vi "Test.vi"() -> ()   [LabVIEW 2019, in "Test.lvlib"]
doc: "This template is for the Queued Message Handler design pattern.\n\nThe Event Handling Loop generates messages based on user interface actions.\n\nThe Message Handling Loop processes messages generated by the Event Handling Loop, or by other messages. The messages are string values, so new messages can be added easily to the Message Cases case structure in the Message Handling Loop. Each message cluster can also provide an optional value for Message Data, which is a variant that can be converted to whatever message-specific data is required.a"
uses:
  Test.lvlib
  Data.ctl
  Message Queue/State Name.ctl
  Support/Message Queue/State Name.ctl
  <vilib>/event_ctls.llb/usereventprio.ctl
  0c61461a-fa07-4497-8c8c-8d3ef654e9c8.vi
  bad579f2-958a-4e04-a1a5-1778729f7708.vi
  681f6a39-68c9-4eb8-ab39-fd2fc03f9966.vi
  <vilib>/Utility/error.llb/Clear Errors.vi
  Message Queue/Enqueue (Single).vi
  <vilib>/Utility/error.llb/Error Cluster From Error Code.vi
  Message Queue/Enqueue (Array).vi
  Support/Message Queue/Reference Queue.vi
  <vilib>/ErrorRing/Error Ring.xnode
  Support/Message Queue/Message Queue.lvlib
panel:
  out "Headline":string
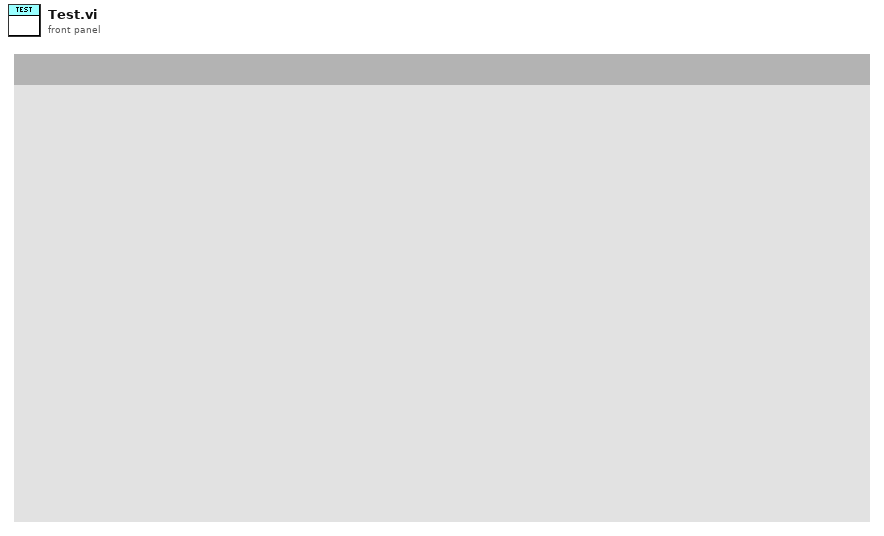
[diagram p1: front panel]
types:
  T1 = typedef "Test.lvlib/State Name.ctl" = enum16{"Default", "Initialize", "Re-Initialize", "Initialize Data", "Initialize Panel", "[Event Structure] Update Data", "Error", "Exit"}
  T2 = typedef "Test.lvlib/Data.ctl" = cluster{"Exit":bool, "States":T1}
  T3 = typedef "Message Queue Ref.ctl" = refnum<queue>
  T4 = typedef "Message Queue.lvlib/State Name.ctl" = enum16{"Default", "Initialize", "Initialize Data", "Initialize Modules", "Initialize Panel", "Close FP", "Open FP", "Initialize Menu", "Mode", "Update Subpanel", "Error", "Open Help", "About", "Open WebResources", "Exit"}
  T5 = typedef "usereventprio.ctl" = enum32{"high priority", "normal priority"}
  T6 = cluster{"Call Chain":string[], "Custom State Name":string, "timed out?":bool}
  T7 = enum16{"Left Button", "Center Button", "Right Button", "Window Close"}
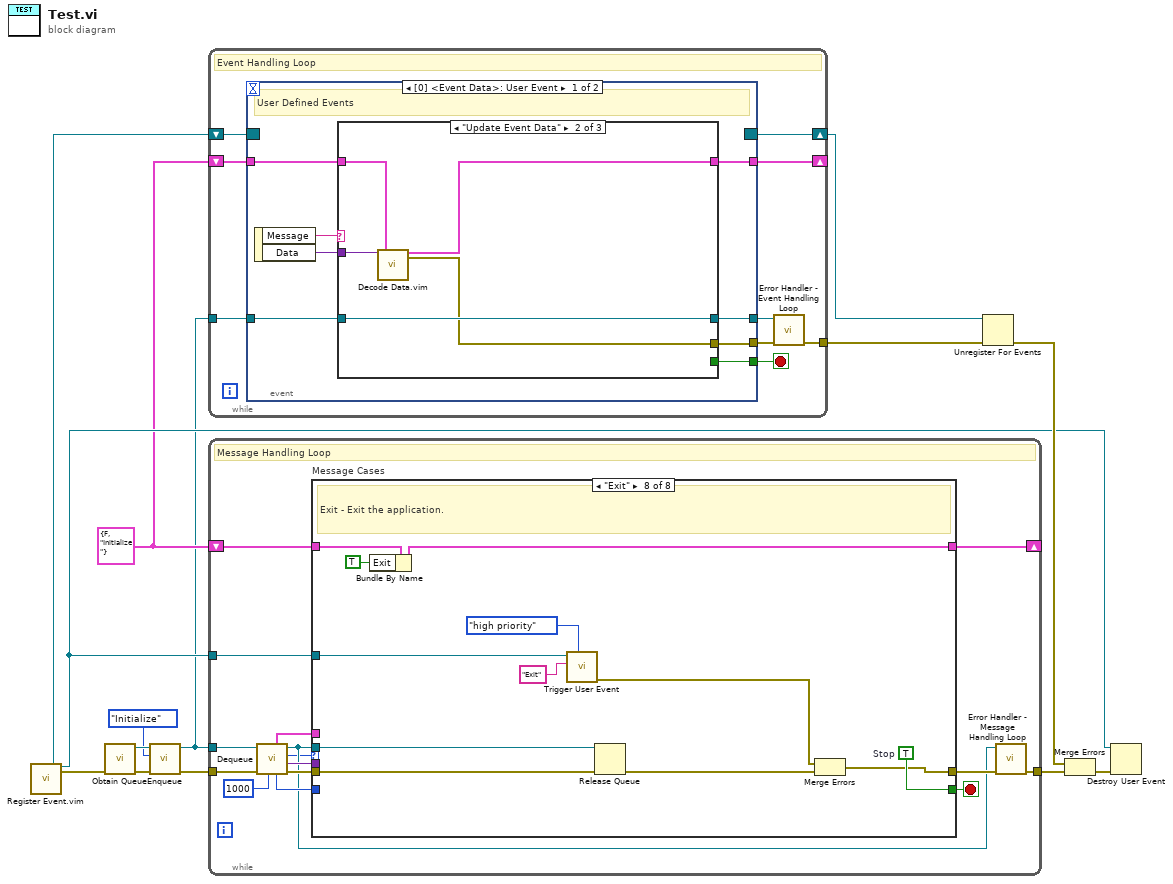
[diagram p0: block diagram]
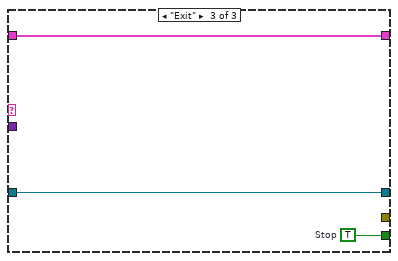
[diagram p3: hidden frame]
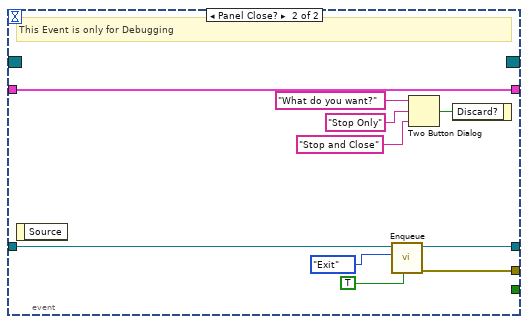
[diagram p4: hidden frame]
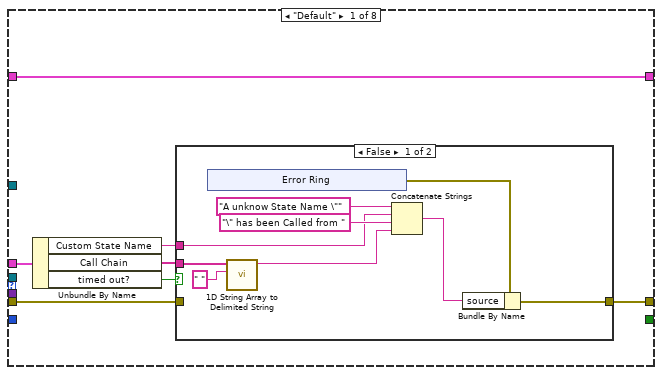
[diagram p5: hidden frame]
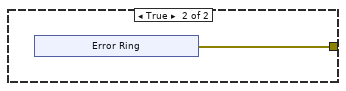
[diagram p6: hidden frame]
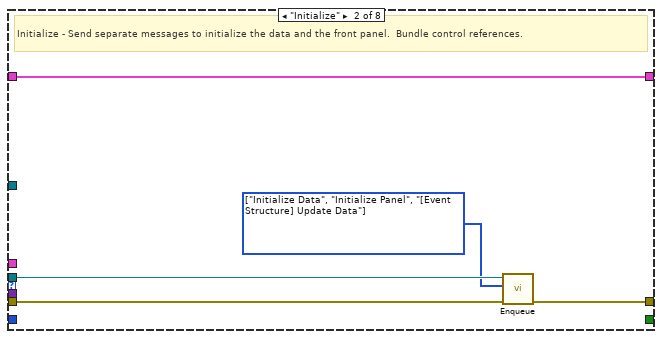
[diagram p7: hidden frame]
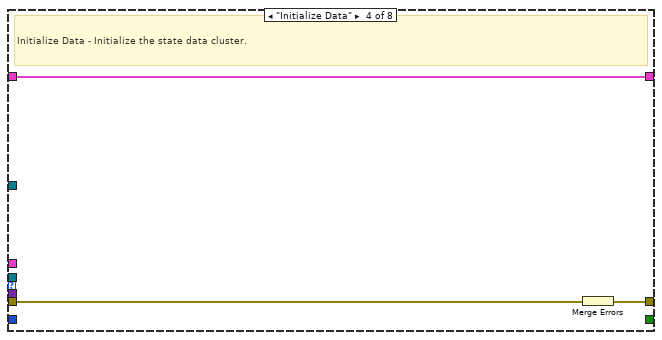
[diagram p9: hidden frame]
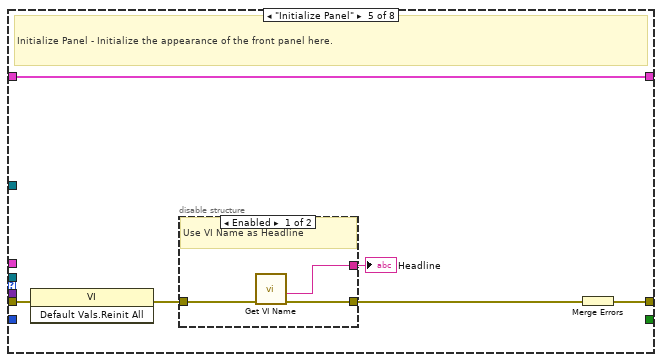
[diagram p10: hidden frame]
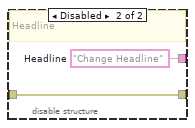
[diagram p11: hidden frame]
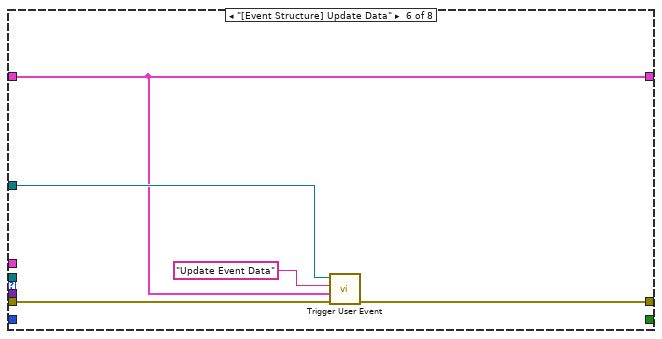
[diagram p12: hidden frame]
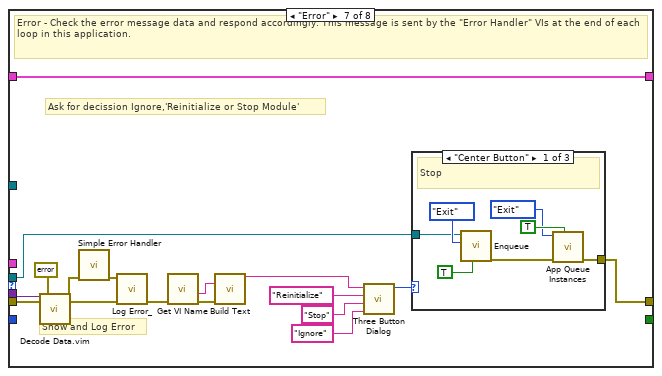
[diagram p13: hidden frame]
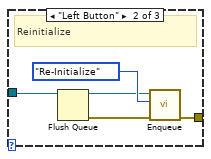
[diagram p14: hidden frame]
diagram:
  w3 = T2 {"Exit"=FALSE, "States"=enum."Initialize"} ("Data")
  n1 = call "Register Event.vim"() -> ("Registration"=w2:refnum<event-registration>, "user event out"=w5:refnum<user-event>, "error out"=w6:errorcluster)  [unwired: 17 in]
  n2 = call "Obtain Queue.vi"("error in (no error)"=w6) -> ("error out"=w10:errorcluster, "Message out"=w11:T3)  [unwired: 9 in]
  n3 = call-poly "Enqueue.vi"("error in (no error)"=w10, "States"=State_Name."Initialize", "Message Queue"=w11) -> ("error out"=w9:errorcluster, "Message Queue dub"=w1:T3)  [unwired: 7 in]
  n4 = while {
    tunnel: w1 -> [w23]
    shift-right: [w15] -> w8
    shift-left: w2 -> [w16]
    tunnel: [w20] -> w12
    shift-right: [w17] -> _
    shift-left: w3 -> [w18]
    stop <- w22 stop-if-true
    # "Event Handling Loop"
    n5 = event shown="[0] <Event Data>: User Event" {
      selector: w16 -> [_ _]
      dyn-events: [_ _] -> w15
      timeout: _ -> [_ _]
      tunnel: [w31 _] -> w22
      tunnel: w23 -> [w28 w44]
      tunnel: [w30 w45] -> w19
      tunnel: [w29 w46] -> w21
      tunnel: w18 -> [w26 w42]
      tunnel: [w27 w42] -> w17
      event User Event {
        # "User Defined Events"
        n6 = event-data() -> ("Message"=w25:string, "Data"=w24:variant)  [unwired: 1 in]
        n7 = case shown="\"Update Event Data\"" w25 {
          tunnel: [_ _ w41] -> w31
          tunnel: [_ w34 _] -> w30
          tunnel: w24 -> [_ w38 _]
          tunnel: [w33 w35 w40] -> w29
          tunnel: w28 -> [w33 w35 w40]
          tunnel: [w32 w36 w39] -> w27
          tunnel: w26 -> [w32 w37 w39]
          frame Default {
          }
          frame "Update Event Data" {
            n8 = call "Decode Data.vim"("Data"=w38, "Type/Default value"=w37) -> ("Data out"=w36:T2, "error out"=w34:errorcluster)  [unwired: 16 in]
          }
          frame "Exit" {
            w41 = TRUE  # Stop
          }
        }
      }
      event Panel Close? {
        # "This Event is only for Debugging"
        n9 = event-data() -> ()  [unwired: 1 in, 1 out]
        n10 = call-poly "Enqueue.vi"("Priority Message? Array"=TRUE ("Priority Message? (F)"), "States"=State_Name."Exit" ("Array"), "Message Queue"=w44) -> ("error out"=w45:errorcluster, "Message Queue dub"=w46:T3)  [unwired: 7 in]
        n11 = Two Button Dialog(message="What do you want?", 1:"Stop and Close" ("F button name (\"Cancel\")"), 2:"Stop Only" ("T button name (\"OK\")")) -> (T button?=w48:bool)
        n12 = event-data("Discard?"=w48) -> ()  [unwired: 1 in, 1 out]
      }
    }
    n13 = call "Error Handler - Event Handling Loop.vi"("error in (no error)"=w19, "Message Queue"=w21) -> ("dup error in"=w20:errorcluster)  [unwired: 8 in, 1 out]
  }
  n14 = while {
    tunnel: w1 -> [w60]
    tunnel: w9 -> [w63]
    tunnel: [w59] -> w14
    shift-right: [w55] -> _
    shift-left: w3 -> [w65]
    tunnel: w5 -> [w54]
    stop <- w64 stop-if-true
    # "Message Handling Loop"
    n15 = call "Dequeue.vi"("timeout in ms (-1)"=1000, "error in (no error)"=w63, "Message Queue"=w60) -> ("error out"=w62:errorcluster, "Message Data"=w61:variant, "State"=w56:T1, "Message Queue dub"=w57:T3, "# elements in queue"=w66:i32, "Caller Info"=w52:T6)  [unwired: 3 in]
    n16 = case "Message Cases" shown="\"Exit\"" w56 {
      tunnel: w57 -> [_ w96 _ _ _ _ w121 w159]
      tunnel: w62 -> [w72 w93 w99 w100 w106 w118 w130 w155]
      tunnel: [w71 w97 w99 w102 w108 w117 w120 w156] -> w58
      tunnel: w65 -> [w73 w95 w98 w101 w107 w115 w135 w154]
      tunnel: [_ _ _ _ _ _ _ w158] -> w64
      tunnel: w61 -> [_ _ _ _ _ _ w127 _]
      tunnel: [w73 w95 w98 w101 w107 w115 w135 w152] -> w55
      tunnel: w54 -> [_ _ _ _ _ w116 _ w151]
      tunnel: w66 -> [_ _ _ _ _ _ _ _]
      tunnel: w52 -> [w70 _ _ _ _ _ _ _]
      frame "Default" {
        n17 = Unbundle By Name(w70) -> ("Custom State Name"=w68:string, "Call Chain"=w69:string[], "timed out?"=w67:bool)
        n18 = case shown="False" w67 {
          tunnel: w72 -> [_ _]
          tunnel: [w80 w87] -> w71
          tunnel: w69 -> [w75 _]
          tunnel: w68 -> [w74 _]
          frame False {
            n19 = xnode "Error Ring"() -> ("error out"=w82:errorcluster)
            n20 = call <vilib>:"1D String Array to Delimited String.vi"("delimiter"=" ", "string array"=w75) -> ("delimited string"=w76:string)  [unwired: 9 in]
            n21 = Concatenate Strings("A unknow State Name \"" ("source"), w74, "\" has been Called from " ("string"), w76) -> (w78:string)
            n22 = Bundle By Name(cluster=w82, "source"=w78) -> (w80:errorcluster)
          }
          frame True {
            n23 = xnode "Error Ring"() -> ("error out"=w87:errorcluster)
          }
        }
      }
      frame "Initialize" {
        w94 = T1[] [enum."Initialize Data", enum."Initialize Panel", enum."[Event Structure] Update Data"] items=["Default", "Initialize", "Re-Initialize", "Initialize Data", "Initialize Panel", "[Event Structure] Update Data", "Error", "Exit"] ("Array")
        # "Initialize - Send separate messages to initialize the data and the front panel.  Bundle control references."
        n24 = call-poly "Enqueue.vi"("error in (no error)"=w93, "States"=w94, "Message Queue"=w96) -> ("error out"=w97:errorcluster)  [unwired: 7 in, 1 out]
      }
      frame "Re-Initialize" {
      }
      frame "Initialize Data" {
        # "Initialize Data - Initialize the state data cluster."
        n25 = Merge Errors(w100) -> (w102:errorcluster)
      }
      frame "Initialize Panel" {
        # "Initialize Panel - Initialize the appearance of the front panel here."
        n26 = invoke class="VI" method="Default Vals.Reinit All"(error in=w106) -> (error out=w105:errorcluster)  [unwired: 2 in, 2 out]
        n27 = disable-structure shown="Enabled" {
          disable-tunnel: w105 -> [w111 w112]
          disable-tunnel: [w110 w112] -> w103
          disable-tunnel: [w109 w113] -> w104
          frame Enabled {
            # "Use VI Name as Headline"
            n28 = call "Get VI Name.vi"("error in (no error)"=w111) -> ("error out"=w110:errorcluster, "VI Name without extension"=w109:string)  [unwired: 8 in, 1 out]
          }
          frame Disabled {
            w113 = "Change Headline"  # Headline
            # "Headline"
          }
        }
        "Headline" <- w104
        n29 = Merge Errors(w103) -> (w108:errorcluster)
      }
      frame "[Event Structure] Update Data" {
        n30 = call "Trigger User Event.vi"("error in (no error)"=w118, "Message Data"=w115, "Message"="Update Event Data", "user event in"=w116) -> ("error out"=w117:errorcluster)  [unwired: 6 in, 1 out]
      }
      frame "Error" {
        # "Ask for decission Ignore,'Reinitialize or Stop Module'"
        # "Show and Log Error"
        # "Error - Check the error message data and respond accordingly. This message is sent by the \"Error Handler\" VIs at the end of each loop in this application."
        n31 = call "Decode Data.vim"("Data"=w127, "error in"=w130, "Type/Default value"=errorcluster {"status"=FALSE, "code"=0, "source"=""} ("error constant")) -> ("Data out"=w128:errorcluster, "error out"=w126:errorcluster)  [unwired: 15 in]
        n32 = call <vilib>:"Simple Error Handler.vi"("error in (no error)"=w128) -> ("error out"=w134:errorcluster)  [unwired: 4 in, 4 out]
        n33 = call "Log Error_.vi"("error in"=w126, "Error log to file"=w134) -> ("error out"=w133:errorcluster)  [unwired: 9 in]
        n34 = call "Get VI Name.vi"("error in (no error)"=w133) -> ("error out"=w131:errorcluster, "VI Name without extension"=w132:string)  [unwired: 8 in, 1 out]
        n35 = call "Build Text"("ModuleName"=w132, "error in (no error)"=w131) -> ("Result"=w119:string)  [unwired: 12 in, 1 out]
        n36 = call <vilib>:"Three Button Dialog.vi"("Right Button Text (\"Cancel\")"="Ignore" ("Right Button Text (\"Cancel\")"), "Center Button Text (\"No\")"="Stop" ("Center Button Text (\"No\")"), "Left Button Text (\"Yes\")"="Reinitialize" ("Left Button Text (\"Yes\")"), "message"=w119) -> ("Which Button?"=w125:T7)  [unwired: 7 in]
        n37 = case shown="\"Center Button\"" w125 {
          tunnel: w121 -> [w137 w143 _]
          tunnel: [w136 w144 _] -> w120
          frame "Center Button" {
            # "Stop"
            n38 = call-poly "Enqueue.vi"("Priority Message? Array"=TRUE ("Priority Message? (F)"), "States"=State_Name."Exit" ("Array"), "Message Queue"=w137) -> ("error out"=w142:errorcluster)  [unwired: 7 in, 1 out]
            n39 = call-poly "App Queue Instances.vi"("Priority Message? (F)"=TRUE, "error in (no error)"=w142, "Tasks"=State_Name."Exit") -> ("error out"=w136:errorcluster)  [unwired: 8 in]
          }
          frame "Left Button" {
            # "Reinitialize"
            n40 = Flush Queue(queue=w143) -> (queue out=w145:T3, error out=w146:errorcluster)  [unwired: 1 in, 1 out]
            n41 = call-poly "Enqueue.vi"("error in (no error)"=w146, "States"=State_Name."Re-Initialize" ("Array"), "Message Queue"=w145) -> ("error out"=w144:errorcluster)  [unwired: 7 in, 1 out]
          }
          frame "Right Button", "Window Close" {
          }
        }
      }
      frame "Exit" {
        w158 = TRUE  # Stop
        # "Exit - Exit the application."
        n42 = Bundle By Name(cluster=w154, "Exit"=TRUE) -> (w152:T2)
        n43 = call "Trigger User Event.vi"("priority (normal)"=usereventprio."high priority", "Message"="Exit", "user event in"=w151) -> ("error out"=w150:errorcluster)  [unwired: 7 in, 1 out]
        n44 = Release Queue(queue=w159, error in (no error)=w155) -> (error out=w157:errorcluster)  [unwired: 1 in, 2 out]
        n45 = Merge Errors(w150, w157) -> (w156:errorcluster)
      }
    }
    n46 = call "Error Handler - Message Handling Loop.vi"("error in (no error)"=w58, "Message Queue"=w57) -> ("dup error in"=w59:errorcluster)  [unwired: 8 in, 1 out]
  }
  n47 = Unregister For Events(event registration refnum=w8, error in=w12) -> (error out=w13:errorcluster)
  n48 = Merge Errors(w13, w14) -> (w7:errorcluster)
  n49 = Destroy User Event(user event=w5, error in=w7) -> ()  [unwired: 1 out]
